vi "Power_Error.vi"   [LabVIEW 2011]
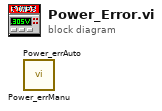
[diagram p0: block diagram]
diagram:
  n1 = call "Power_errManu.vi"() -> ()  [unwired: 5 in, 2 out]
  n2 = call "Power_errAuto.vi"() -> ()  [unwired: 4 in, 3 out]
